vi "Initialize.vi"(8 "error in (no error)":errorcluster caption="错误输入（无错误）", 9 "外观":cluster{"小数位数":u8, "字体颜色":u32, "背景颜色":u32}, 10 "引用":T1, 11 "DigitalDisplay 输入":refnum<class "DigitalDisplay.lvclass">) -> (0 "error out":errorcluster caption="错误输出", 3 "DigitalDisplay 输出":refnum<class "DigitalDisplay.lvclass">)   [LabVIEW 2018, in "DataDisplay.lvlib" / "DigitalDisplay.lvclass"]
uses:
  DigitalDisplay.lvclass
  DigitalDisplayRef.ctl
  TypeDefine/DD_DataStream.ctl
  DigitalDisplay.lvclass/DigitalDisplay.ctl
  DataDisplay.lvlib
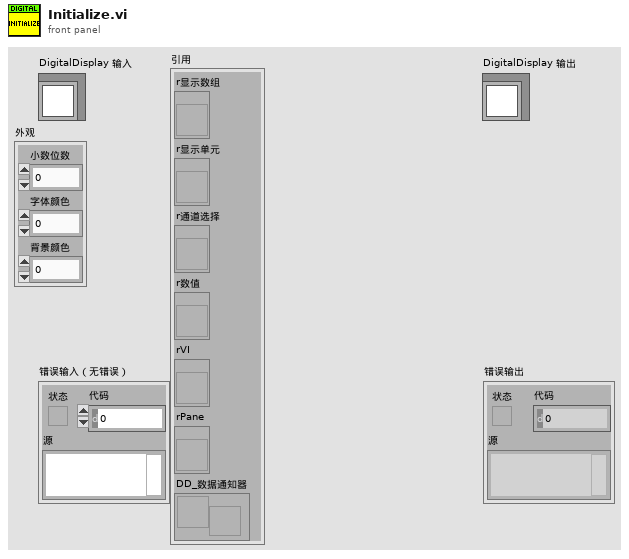
[diagram p1: front panel]
types:
  T1 = typedef "DataDisplay.lvlib/DigitalDisplay.lvclass/DigitalDisplayRef.ctl" = cluster{"r显示数组":refnum<vi>, "r显示单元":refnum<vi>, "r通道选择":refnum<vi>, "r数值":refnum<vi>, "rVI":refnum<vi>, "rPane":refnum<vi>, "DD_数据通知器":refnum<notifier>}
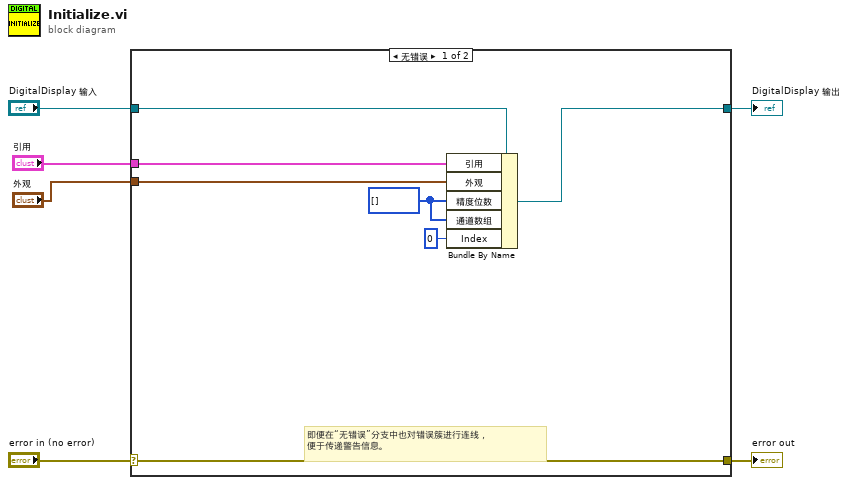
[diagram p0: block diagram]
diagram:
  n1 = case shown="无错误" "error in (no error)" {
    selector: "error in (no error)" -> [w12 w15]
    tunnel: [w12 w15] -> w5
    tunnel: [w11 w14] -> w3
    tunnel: "DigitalDisplay 输入" -> [w13 w14]
    tunnel: "外观" -> [w10 _]
    tunnel: "引用" -> [w7 _]
    frame No Error {
      w9 = i32[] [] ("精度位数")
      # "即便在“无错误”分支中也对错误簇进行连线，\n便于传递警告信息。"
      n2 = Bundle By Name(cluster=w13, "引用"=w7, "外观"=w10, "精度位数"=w9, "通道数组"=w9, "Index"=0) -> (w11:refnum<class "DigitalDisplay.lvclass">)
    }
    frame Error {
    }
  }
  "error out" <- w5
  "DigitalDisplay 输出" <- w3
